vi "Initialize TCP.vi"(7 "timeout, ms (1000)":u32=1000, 8 "error in (no error)":errorcluster, 10 "port (8000)":u16=8000, 11 "ip address":string) -> (0 "error out":errorcluster, 3 "VGC out":refnum<class "PL Inficon VGC.lvclass">)   [LabVIEW 2015, in "PL Inficon VGC.lvclass"]
doc: "Initializes connection to device using specified settings."
uses:
  PL Inficon VGC.lvclass
  PL Inficon VGC.lvclass/PL Inficon VGC.ctl
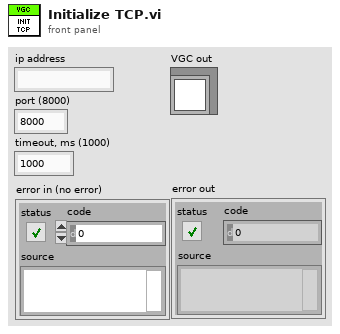
[diagram p1: front panel]
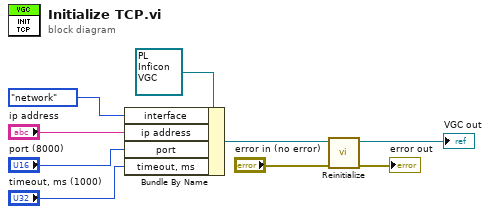
[diagram p0: block diagram]
diagram:
  n1 = Bundle By Name(cluster=refnum<class "PL Inficon VGC.lvclass"> refnum, "interface"=enum16{"serial", "network"}."network", "ip address"="ip address", "port"="port (8000)", "timeout, ms"="timeout, ms (1000)") -> (w9:refnum<class "PL Inficon VGC.lvclass">)
  n2 = call "Reinitialize.vi"("error in (no error)"="error in (no error)", "VGC in"=w9) -> ("error out"=→"error out":errorcluster, "VGC out"=→"VGC out":refnum<class "PL Inficon VGC.lvclass">)  [unwired: 8 in]
